vi "Func-엑셀 데이터를 그래프로 출력.vi"() -> ()   [LabVIEW 2015] (continued)
303.91\n303.93\n303.94\n303.96\n303.98\n303.99\n304.01\n304.03\n304.04\n304.06\n304.08\n304.1\n304.11\n304.13\n304.14\n304.16\n304.18\n304.19\n304.21\n304.23\n304.24\n304.26\n304.28\n304.3\n304.31\n304.33\n304.34\n304.36\n304.38\n304.39\n304.41\n304.43\n304.44\n304.46\n304.48\n304.49\n304.51\n304.53\n304.54\n304.56\n304.58\n304.59\n304.61\n304.63\n304.64\n304.66\n304.68\n304.69\n304.71\n304.73\n304.74\n304.76\n304.78\n304.79\n304.81\n304.83\n304.84\n304.86\n304.88\n304.89\n304.91\n304.93\n304.94\n304.96\n304.98\n304.99\n305.01\n305.03\n305.04\n305.06\n305.08\n305.09\n305.11\n305.13\n305.14\n305.16\n305.18\n305.19\n305.21\n305.23\n305.24\n305.26\n305.28\n305.29\n305.31\n305.33\n305.34\n305.36\n305.38\n305.39\n305.41\n305.43\n305.44\n305.46\n305.48\n305.49\n305.51\n305.53\n305.54\n305.56\n305.58\n305.59\n305.61\n305.63\n305.64\n305.66\n305.68\n305.69\n305.71\n305.73\n305.74\n305.76\n305.78\n305.79\n305.81\n305.83\n305.84\n305.86\n305.88\n305.89\n305.91\n305.93\n305.94\n305.96\n305.98\n305.99\n306.01\n306.03\n306.04\n306.06\n306.08\n306.09\n306.11\n306.13\n306.15\n306.16\n306.18\n306.19\n306.21\n306.23\n306.25\n306.26\n306.28\n306.29\n306.31\n306.33\n306.34\n306.36\n306.38\n306.39\n306.41\n306.43\n306.44\n306.46\n306.48\n306.5\n306.51\n306.53\n306.54\n306.56\n306.58\n306.6\n306.61\n306.63\n306.64\n306.66\n306.68\n306.69\n306.71\n306.73\n306.74\n306.76\n306.78\n306.79\n306.81\n306.83\n306.84\n306.86\n306.88\n306.89\n306.91\n306.93\n306.95\n306.96\n306.98\n306.99\n307.01\n307.03\n307.04\n307.06\n307.08\n307.09\n307.11\n307.13\n307.14\n307.16\n307.18\n307.2\n307.21\n307.23\n307.24\n307.26\n307.28\n307.29\n307.31\n307.33\n307.34\n307.36\n307.38\n307.39\n307.41\n307.43\n307.44\n307.46\n307.48\n307.49\n307.51\n307.53\n307.54\n307.56\n307.58\n307.59\n307.61\n307.63\n307.65\n307.66\n307.68\n307.69\n307.71\n307.73\n307.74\n307.76\n307.78\n307.79\n307.81\n307.83\n307.84\n307.86\n307.88\n307.89\n307.91\n307.93\n307.94\n307.96\n307.98\n307.99\n308.01\n308.03\n308.04\n308.06\n308.08\n308.09\n308.11\n308.13\n308.14\n308.16\n308.18\n308.19\n308.21\n308.23\n308.24\n308.26\n308.28\n308.29\n308.31\n308.33\n308.34\n308.36\n308.38\n308.39\n308.41\n308.43\n308.44\n308.46\n308.48\n308.49\n308.51\n308.53\n308.54\n308.56\n308.58\n308.59\n308.61\n308.63\n308.64\n308.66\n308.68\n308.69\n308.71\n308.73\n308.74\n308.76\n308.78\n308.79\n308.81\n308.83\n308.84\n308.86\n308.88\n308.89\n308.91\n308.93\n308.94\n308.96\n308.98\n309\n309.01\n309.03\n309.04\n309.06\n309.08\n309.09\n309.11\n309.13\n309.14\n309.16\n309.18\n309.19\n309.21\n309.23\n309.25\n309.26\n309.28\n309.29\n309.31\n309.33\n309.35\n309.36\n309.38\n309.39\n309.41\n309.43\n309.44\n309.46\n309.48\n309.49\n309.51\n309.53\n309.54\n309.56\n309.58\n309.6\n309.61\n309.63\n309.64\n309.66\n309.68\n309.7\n309.71\n309.73\n309.74\n309.76\n309.78\n309.8\n309.81\n309.83\n309.84\n309.86\n309.88\n309.89\n309.91\n309.93\n309.94\n309.96\n309.98\n309.99\n310.01\n310.03\n310.04\n310.06\n310.08\n310.09\n310.11\n310.13\n310.14\n310.16\n310.18\n310.19\n310.21\n310.23\n310.24\n310.26\n310.28\n310.3\n310.31\n310.33\n310.34\n310.36\n310.38\n310.39\n310.41\n310.43\n310.44\n310.46\n310.48\n310.49\n310.51\n310.53\n310.54\n310.56\n310.58\n310.59\n310.61\n310.63\n310.64\n310.66\n310.68\n310.69\n310.71\n310.73\n310.74\n310.76\n310.78\n310.79\n310.81\n310.83\n310.84\n310.86\n310.88\n310.89\n310.91\n310.93\n310.94\n310.96\n310.98\n310.99\n311.01\n311.03\n311.04\n311.06\n311.08\n311.09\n311.11\n311.13\n311.14\n311.16\n311.18\n311.19\n311.21\n311.23\n311.24\n311.26\n311.28\n311.29\n311.31\n311.33\n311.34\n311.36\n311.38\n311.39\n311.41\n311.43\n311.44\n311.46\n311.48\n311.49\n311.51\n311.53\n311.54\n311.56\n311.58\n311.59\n311.61\n311.63\n311.64\n311.66\n311.68\n311.69\n311.71\n311.73\n311.74\n311.76\n311.78\n311.79\n311.81\n311.83\n311.84\n311.86\n311.88\n311.89\n311.91\n311.93\n311.94\n311.96\n311.98\n311.99\n312.01\n312.03\n312.04\n312.06\n312.08\n312.1\n312.11\n312.13\n312.14\n312.16\n312.18\n312.19\n312.21\n312.23\n312.24\n312.26\n312.28\n312.29\n312.31\n312.33\n312.35\n312.36\n312.38\n312.39\n312.41\n312.43\n312.44\n312.46\n312.48\n312.49\n312.51\n312.53\n312.54\n312.56\n312.58\n312.59\n312.61\n312.63\n312.64\n312.66\n312.68\n312.7\n312.71\n312.73\n312.74\n312.76\n312.78\n312.8\n312.81\n312.83\n312.84\n312.86\n312.88\n312.89\n312.91\n312.93\n312.94\n312.96\n312.98\n312.99\n313.01\n313.03\n313.05\n313.06\n313.08\n313.09\n313.11\n313.13\n313.14\n313.16\n313.18\n313.19\n313.21\n313.23\n313.24\n313.26\n313.28\n313.29\n313.31\n313.33\n313.34\n313.36\n313.38\n313.39\n313.41\n313.43\n313.44\n313.46\n313.48\n313.49\n313.51\n313.53\n313.54\n313.56\n313.58\n313.59\n313.61\n313.63\n313.64\n313.66\n313.68\n313.69\n313.71\n313.73\n313.75\n313.76\n313.78\n313.79\n313.81\n313.83\n313.84\n313.86\n313.88\n313.89\n313.91\n313.93\n313.94\n313.96\n313.98\n313.99\n314.01\n314.03\n314.04\n314.06\n314.08\n314.09\n314.11\n314.13\n314.14\n314.16\n314.18\n314.19\n314.21\n314.23\n314.24\n314.26\n314.28\n314.29\n314.31\n314.33\n314.34\n314.36\n314.38\n314.39\n314.41\n314.43\n314.44\n314.46\n314.48\n314.49\n314.51\n314.53\n314.54\n314.56\n314.58\n314.59\n314.61\n314.63\n314.64\n314.66\n314.68\n314.69\n314.71\n314.73\n314.74\n314.76\n314.78\n314.79\n314.81\n314.83\n314.84\n314.86\n314.88\n314.89\n314.91\n314.93\n314.94\n314.96\n314.98\n314.99\n315.01\n315.03\n315.04\n315.06\n315.08\n315.09\n315.11\n315.13\n315.14\n315.16\n315.18\n315.19\n315.21\n315.23\n315.24\n315.26\n315.28\n315.29\n315.31\n315.33\n315.34\n315.36\n315.38\n315.39\n315.41\n315.43\n315.45\n315.46\n315.48\n315.49\n315.51\n315.53\n315.55\n315.56\n315.58\n315.59\n315.61\n315.63\n315.64\n315.66\n315.68\n315.69\n315.71\n315.73\n315.74\n315.76\n315.78\n315.8\n315.81\n315.83\n315.84\n315.86\n315.88\n315.9\n315.91\n315.93\n315.94\n315.96\n315.98\n315.99\n316.01\n316.03\n316.04\n316.06\n316.08\n316.09\n316.11\n316.13\n316.14\n316.16\n316.18\n316.19\n316.21\n316.23\n316.24\n316.26\n316.28\n316.29\n316.31\n316.33\n316.35\n316.36\n316.38\n316.39\n316.41\n316.43\n316.44\n316.46\n316.48\n316.49\n316.51\n316.53\n316.54\n316.56\n316.58\n316.59\n316.61\n316.63\n316.64\n316.66\n316.68\n316.7\n316.71\n316.73\n316.74\n316.76\n316.78\n316.79\n316.81\n316.83\n316.84\n316.86\n316.88\n316.89\n316.91\n316.93\n316.94\n316.96\n316.98\n316.99\n317.01\n317.03\n317.04\n317.06\n317.08\n317.09\n317.11\n317.13\n317.14\n317.16\n317.18\n317.19\n317.21\n317.23\n317.24\n317.26\n317.28\n317.29\n317.31\n317.33\n317.34\n317.36\n317.38\n317.39\n317.41\n317.43\n317.44\n317.46\n317.48\n317.49\n317.51\n317.53\n317.54\n317.56\n317.58\n317.59\n317.61\n317.63\n317.64\n317.66\n317.68\n317.69\n317.71\n317.73\n317.74\n317.76\n317.78\n317.79\n317.81\n317.83\n317.84\n317.86\n317.88\n317.89\n317.91\n317.93\n317.94\n317.96\n317.98\n317.99\n318.01\n318.03\n318.04\n318.06\n318.08\n318.09\n318.11\n318.13\n318.14\n318.16\n318.18\n318.19\n318.21\n318.23\n318.24\n318.26\n318.28\n318.3\n318.31\n318.33\n318.34\n318.36\n318.38\n318.39\n318.41\n318.43\n318.44\n318.46\n318.48\n318.49\n318.51\n318.53\n318.54\n318.56\n318.58\n318.59\n318.61\n318.63\n318.64\n318.66\n318.68\n318.69\n318.71\n318.73\n318.74\n318.76\n318.78\n318.79\n318.81\n318.83\n318.84\n318.86\n318.88\n318.9\n318.91\n318.93\n318.94\n318.96\n318.98\n319\n319.01\n319.03\n319.04\n319.06\n319.08\n319.09\n319.11\n319.13\n319.14\n319.16\n319.18\n319.19\n319.21\n319.23\n319.24\n319.26\n319.28\n319.29\n319.31\n319.33\n319.34\n319.36\n319.38\n319.39\n319.41\n319.43\n319.44\n319.46\n319.48\n319.5\n319.51\n319.53\n319.54\n319.56\n319.58\n319.59\n319.61\n319.63\n319.64\n319.66\n319.68\n319.7\n319.71\n319.73\n319.74\n319.76\n319.78\n319.8\n319.81\n319.83\n319.84\n319.86\n319.88\n319.89\n319.91\n319.93\n319.94\n319.96\n319.98\n319.99\n320.01\n320.03\n320.04\n320.06\n320.08\n320.1\n320.11\n320.13\n320.14\n320.16\n320.18\n320.19\n320.21\n320.23\n320.24\n320.26\n320.28\n320.29\n320.31\n320.33\n320.34\n320.36\n320.38\n320.39\n320.41\n320.43\n320.44\n320.46\n320.48\n320.49\n320.51\n320.53\n320.54\n320.56\n320.58\n320.59\n320.61\n320.63\n320.64\n320.66\n320.68\n320.69\n320.71\n320.73\n320.74\n320.76\n320.78\n320.79\n320.81\n320.83\n320.84\n320.86\n320.88\n320.89\n320.91\n320.93\n320.94\n320.96\n320.98\n320.99\n321.01\n321.03\n321.04\n321.06\n321.08\n321.09\n321.11\n321.13\n321.14\n321.16\n321.18\n321.19\n321.21\n321.23\n321.24\n321.26\n321.28\n321.3\n321.31\n321.33\n321.34\n321.36\n321.38\n321.39\n321.41\n321.43\n321.44\n321.46\n321.48\n321.49\n321.51\n321.53\n321.54\n321.56\n321.58\n321.59\n321.61\n321.63\n321.65\n321.66\n321.68\n321.69\n321.71\n321.73\n321.75\n321.76\n321.78\n321.79\n321.81\n321.83\n321.84\n321.86\n321.88\n321.89\n321.91\n321.93\n321.94\n321.96\n321.98\n322\n322.01\n322.03\n322.04\n322.06\n322.08\n322.1\n322.11\n322.13\n322.14\n322.16\n322.18\n322.19\n322.21\n322.23\n322.24\n322.26\n322.28\n322.29\n322.31\n322.33\n322.35\n322.36\n322.38\n322.39\n322.41\n322.43\n322.44\n322.46\n322.48\n322.49\n322.51\n322.53\n322.54\n322.56\n322.58\n322.6\n322.61\n322.63\n322.64\n322.66\n322.68\n322.69\n322.71\n322.73\n322.74\n322.76\n322.78\n322.79\n322.81\n322.83\n322.84\n322.86\n322.88\n322.89\n322.91\n322.93\n322.94\n322.96\n322.98\n322.99\n323.01\n323.03\n323.04\n323.06\n323.08\n323.09\n323.11\n323.13\n323.14\n323.16\n323.18\n323.19\n323.21\n323.23\n323.24\n323.26\n323.28\n323.29\n323.31\n323.33\n323.34\n323.36\n323.38\n323.39\n323.41\n323.43\n323.44\n323.46\n323.48\n323.49\n323.51\n323.53\n323.54\n323.56\n323.58\n323.59\n323.61\n323.63\n323.64\n323.66\n323.68\n323.69\n323.71\n323.73\n323.74\n323.76\n323.78\n323.79\n323.81\n323.83\n323.84\n323.86\n323.88\n323.89\n323.91\n323.93\n323.94\n323.96\n323.98\n323.99\n324.01\n324.03\n324.04\n324.06\n324.08\n324.09\n324.11\n324.13\n324.14\n324.16\n324.18\n324.19\n324.21\n324.23\n324.24\n324.26\n324.28\n324.29\n324.31\n324.33\n324.34\n324.36\n324.38\n324.39\n324.41\n324.43\n324.44\n324.46\n324.48\n324.49\n324.51\n324.53\n324.54\n324.56\n324.58\n324.59\n324.61\n324.63\n324.64\n324.66\n324.68\n324.69\n324.71\n324.73\n324.75\n324.76\n324.78\n324.79\n324.81\n324.83\n324.85\n324.86\n324.88\n324.89\n324.91\n324.93\n324.94\n324.96\n324.98\n324.99\n325.01\n325.03\n325.04\n325.06\n325.08\n325.1\n325.11\n325.13\n325.14\n325.16\n325.18\n325.2\n325.21\n325.23\n325.24\n325.26\n325.28\n325.29\n325.31\n325.33\n325.34\n325.36\n325.38\n325.39\n325.41\n325.43\n325.45\n325.46\n325.48\n325.49\n325.51\n325.53\n325.55\n325.56\n325.58\n325.59\n325.61\n325.63\n325.64\n325.66\n325.68\n325.7\n325.71\n325.73\n325.74\n325.76\n325.78\n325.8\n325.81\n325.83\n325.84\n325.86\n325.88\n325.9\n325.91\n325.93\n325.94\n325.96\n325.98\n325.99\n326.01\n326.03\n326.04\n326.06\n326.08\n326.09\n326.11\n326.13\n326.14\n326.16\n326.18\n326.19\n326.21\n326.23\n326.24\n326.26\n326.28\n326.29\n326.31\n326.33\n326.34\n326.36\n326.38\n326.39\n326.41\n326.43\n326.44\n326.46\n326.48\n326.49\n326.51\n326.53\n326.54\n326.56\n326.58\n326.59\n326.61\n326.63\n326.64\n326.66\n326.68\n326.69\n326.71\n326.73\n326.74\n326.76\n326.78\n326.79\n326.81\n326.83\n326.84\n326.86\n326.88\n326.89\n326.91\n326.93\n326.94\n326.96\n326.98\n326.99\n327.01\n327.03\n327.04\n327.06\n327.08\n327.09\n327.11\n327.13\n327.14\n327.16\n327.18\n327.19\n327.21\n327.23\n327.24\n327.26\n327.28\n327.29\n327.31\n327.33\n327.34\n327.36\n327.38\n327.39\n327.41\n327.43\n327.44\n327.46\n327.48\n327.49\n327.51\n327.53\n327.54\n327.56\n327.58\n327.59\n327.61\n327.63\n327.64\n327.66\n327.68\n327.69\n327.71\n327.73\n327.74\n327.76\n327.78\n327.79\n327.81\n327.83\n327.85\n327.86\n327.88\n327.89\n327.91\n327.93\n327.94\n327.96\n327.98\n327.99\n328.01\n328.03\n328.04\n328.06\n328.08\n328.09\n328.11\n328.13\n328.14\n328.16\n328.18\n328.2\n328.21\n328.23\n328.24\n328.26\n328.28\n328.3\n328.31\n328.33\n328.34\n328.36\n328.38\n328.39\n328.41\n328.43\n328.44\n328.46\n328.48\n328.49\n328.51\n328.53\n328.55\n328.56\n328.58\n328.59\n328.61\n328.63\n328.64\n328.66\n328.68\n328.69\n328.71\n328.73\n328.74\n328.76\n328.78\n328.8\n328.81\n328.83\n328.84\n328.86\n328.88\n328.9\n328.91\n328.93\n328.94\n328.96\n328.98\n328.99\n329.01\n329.03\n329.04\n329.06\n329.08\n329.1\n329.11\n329.13\n329.15\n329.16\n329.18\n329.19\n329.21\n329.23\n329.24\n329.26\n329.28\n329.29\n329.31\n329.33\n329.34\n329.36\n329.38\n329.39\n329.41\n329.43\n329.45\n329.46\n329.48\n329.49\n329.51\n329.53\n329.54\n329.56\n329.58\n329.59\n329.61\n329.63\n329.64\n329.66\n329.68\n329.69\n329.71\n329.73\n329.74\n329.76\n329.78\n329.79\n329.81\n329.83\n329.84\n329.86\n329.88\n329.89\n329.91\n329.93\n329.94\n329.96\n329.98\n329.99\n330.01\n330.03\n330.04\n330.06\n330.08\n330.09\n330.11\n330.13\n330.14\n330.16\n330.18\n330.19\n330.21\n330.23\n330.24\n330.26\n330.28\n330.29\n330.31\n330.33\n330.34\n330.36\n330.38\n330.39\n330.41\n330.43\n330.44\n330.46\n330.48\n330.49\n330.51\n330.53\n330.54\n330.56\n330.58\n330.6\n330.61\n330.63\n330.64\n330.66\n330.68\n330.69\n330.71\n330.73\n330.74\n330.76\n330.78\n330.79\n330.81\n330.83\n330.84\n330.86\n330.88\n330.89\n330.91\n330.93\n330.95\n330.96\n330.98\n330.99\n331.01\n331.03\n331.05\n331.06\n331.08\n331.09\n331.11\n331.13\n331.14\n331.16\n331.18\n331.19\n331.21\n331.23\n331.24\n331.26\n331.28\n331.3\n331.31\n331.33\n331.34\n331.36\n331.38\n331.4\n331.41\n331.43\n331.44\n331.46\n331.48\n331.49\n331.51\n331.53\n331.54\n331.56\n331.58\n331.59\n331.61\n331.63\n331.65\n331.66\n331.68\n331.69\n331.71\n331.73\n331.74\n331.76\n331.78\n331.79\n331.81\n331.83\n331.84\n331.86\n331.88\n331.9\n331.91\n331.93\n331.94\n331.96\n331.98\n332\n332.01\n332.03\n332.04\n332.06\n332.08\n332.09\n332.11\n332.13\n332.14\n332.16\n332.18\n332.19\n332.21\n332.23\n332.25\n332.26\n332.28\n332.29\n332.31\n332.33\n332.34\n332.36\n332.38\n332.39\n332.41\n332.43\n332.45\n332.46\n332.48\n332.49\n332.51\n332.53\n332.54\n332.56\n332.58\n332.59\n332.61\n332.63\n332.64\n332.66\n332.68\n332.69\n332.71\n332.73\n332.74\n332.76\n332.78\n332.79\n332.81\n332.83\n332.84\n332.86\n332.88\n332.89\n332.91\n332.93\n332.94\n332.96\n332.98\n332.99\n333.01\n333.03\n333.04\n333.06\n333.08\n333.09\n333.11\n333.13\n333.14\n333.16\n333.18\n333.19\n333.21\n333.23\n333.24\n333.26\n333.28\n333.29\n333.31\n333.33\n333.34\n333.36\n333.38\n333.39\n333.41\n333.43\n333.44\n333.46\n333.48\n333.49\n333.51\n333.53\n333.54\n333.56\n333.58\n333.59\n333.61\n333.63\n333.64\n333.66\n333.68\n333.69\n333.71\n333.73\n333.74\n333.76\n333.78\n333.79\n333.81\n333.83\n333.84\n333.86\n333.88\n333.89\n333.91\n333.93\n333.94\n333.96\n333.98\n333.99\n334.01\n334.03\n334.05\n334.06\n334.08\n334.09\n334.11\n334.13\n334.14\n334.16\n334.18\n334.19\n334.21\n334.23\n334.24\n334.26\n334.28\n334.29\n334.31\n334.33\n334.34\n334.36\n334.38\n334.4\n334.41\n334.43\n334.44\n334.46\n334.48\n334.5\n334.51\n334.53\n334.54\n334.56\n334.58\n334.59\n334.61\n334.63\n334.64\n334.66\n334.68\n334.69\n334.71\n334.73\n334.75\n334.76\n334.78\n334.79\n334.81\n334.83\n334.85\n334.86\n334.88\n334.89\n334.91\n334.93\n334.94\n334.96\n334.98\n334.99\n335.01\n335.03\n335.04\n335.06\n335.08\n335.1\n335.11\n335.13\n335.14\n335.16\n335.18\n335.2\n335.21\n335.23\n335.24\n335.26\n335.28\n335.3\n335.31\n335.33\n335.34\n335.36\n335.38\n335.39\n335.41\n335.43\n335.45\n335.46\n335.48\n335.49\n335.51\n335.53\n335.54\n335.56\n335.58\n335.59\n335.61\n335.63\n335.64\n335.66\n335.68\n335.69\n335.71\n335.73\n335.74\n335.76\n335.78\n335.79\n335.81\n335.83\n335.84\n335.86\n335.88\n335.89\n335.91\n335.93\n335.94\n335.96\n335.98\n335.99\n336.01\n336.03\n336.04\n336.06\n336.08\n336.09\n336.11\n336.13\n336.14\n336.16\n336.18\n336.19\n336.21\n336.23\n336.24\n336.26\n336.28\n336.29\n336.31\n336.33\n336.34\n336.36\n336.38\n336.39\n336.41\n336.43\n336.44\n336.46\n336.48\n336.49\n336.51\n336.53\n336.54\n336.56\n336.58\n336.59\n336.61\n336.63\n336.64\n336.66\n336.68\n336.69\n336.71\n336.73\n336.74\n336.76\n336.78\n336.79\n336.81\n336.83\n336.84\n336.86\n336.88\n336.89\n336.91\n336.93\n336.94\n336.96\n336.98\n336.99\n337.01\n337.03\n337.04\n337.06\n337.08\n337.09\n337.11\n337.13\n337.14\n337.16\n337.18\n337.19\n337.21\n337.23\n337.25\n337.26\n337.28\n337.29\n337.31\n337.33\n337.34\n337.36\n337.38\n337.39\n337.41\n337.43\n337.44\n337.46\n337.48\n337.5\n337.51\n337.53\n337.54\n337.56\n337.58\n337.6\n337.61\n337.63\n337.64\n337.66\n337.68\n337.69\n337.71\n337.73\n337.74\n337.76\n337.78\n337.79\n337.81\n337.83\n337.85\n337.86\n337.88\n337.89\n337.91\n337.93\n337.95\n337.96\n337.98\n337.99\n338.01\n338.03\n338.04\n338.06\n338.08\n338.1\n338.11\n338.13\n338.14\n338.16\n338.18\n338.2\n338.21\n338.23\n338.24\n338.26\n338.28\n338.29\n338.31\n338.33\n338.34\n338.36\n338.38\n338.39\n338.41\n338.43\n338.44\n338.46\n338.48\n338.49\n338.51\n338.53\n338.55\n338.56\n338.58\n338.59\n338.61\n338.63\n338.64\n338.66\n338.68\n338.69\n338.71\n338.73\n338.74\n338.76\n338.78\n338.79\n338.81\n338.83\n338.84\n338.86\n338.88\n338.89\n338.91\n338.93\n338.94\n338.96\n338.98\n338.99\n339.01\n339.03\n339.04\n339.06\n339.08\n339.09\n339.11\n339.13\n339.14\n339.16\n339.18\n339.19\n339.21\n339.23\n339.24\n339.26\n339.28\n339.29\n339.31\n339.33\n339.34\n339.36\n339.38\n339.39\n339.41\n339.43\n339.44\n339.46\n339.48\n339.49\n339.51\n339.53\n339.54\n339.56\n339.58\n339.59\n339.61\n339.63\n339.64\n339.66\n339.68\n339.69\n339.71\n339.73\n339.74\n339.76\n339.78\n339.79\n339.81\n339.83\n339.84\n339.86\n339.88\n339.89\n339.91\n339.93\n339.94\n339.96\n339.98\n339.99\n340.01\n340.03\n340.04\n340.06\n340.08\n340.09\n340.11\n340.13\n340.14\n340.16\n340.18\n340.19\n340.21\n340.23\n340.24\n340.26\n340.28\n356.83\n357\n357.16\n357.33\n357.5\n357.66\n357.83\n358\n358.16\n358.33\n358.5\n358.66\n358.83\n359\n359.16\n359.33\n359.5\n359.67\n359.83\n360\n360.16\n360.33\n360.51\n360.67\n360.84\n361.01\n361.17\n361.34\n361.51\n361.67\n361.84\n362.01\n362.17\n362.34\n362.51\n362.67\n362.84\n363.01\n363.17\n363.34\n363.51\n363.67\n363.84\n364.01\n364.17\n364.34\n364.51\n364.67\n364.84\n365.01\n365.17\n365.34\n365.51\n365.67\n365.84\n366.01\n366.17\n366.34\n366.51\n366.67\n366.84\n367.01\n367.18\n367.35\n367.51\n367.68\n367.85\n368.01\n368.18\n368.35\n368.52\n368.68\n368.85\n369.01\n369.18\n369.35\n369.51\n369.68\n369.85\n370.01\n370.18\n370.35\n370.51\n370.68\n370.85\n371.01\n371.18\n371.35\n371.51\n371.68\n371.85\n372.01\n372.18\n372.35\n372.51\n372.68\n372.85\n373.01\n373.18\n373.35\n373.51\n373.68\n373.85\n374.01\n374.18\n374.35\n374.51\n374.68\n374.85\n375.01\n375.18\n375.35\n375.52\n375.68\n375.85\n376.01\n376.18\n376.35\n376.51\n376.68\n376.85\n377.01\n377.18\n377.35\n377.51\n377.68\n377.85\n378.01\n378.18\n378.35\n378.51\n378.68\n378.85\n379.01\n379.2\n379.35\n379.51\n379.68\n379.85\n380.01\n380.2\n380.37\n380.53\n380.7\n380.85\n381.03\n381.2\n381.37\n381.53\n381.7\n381.87\n382.03\n382.2\n382.37\n382.53\n382.7\n382.87\n383.04\n383.19\n383.36\n383.52\n383.69\n383.86\n384.02\n384.19\n384.36\n384.52\n384.69\n384.86\n385.02\n385.19\n385.36\n385.52\n385.69\n385.86\n386.02\n386.19\n386.36\n386.52\n386.69\n386.86\n387.02\n387.19\n387.36\n387.52\n387.69\n387.86\n388.02\n388.19\n388.36\n388.52\n388.69\n388.86\n389.02\n389.19\n389.36\n389.52\n389.69\n389.86\n390.02\n390.19\n390.36\n390.52\n390.69\n390.86\n391.02\n391.19\n391.36\n391.52\n391.69\n391.86\n392.02\n392.19\n392.36\n392.52\n392.69\n392.86\n393.02\n393.19\n393.36\n393.52\n393.69\n393.86\n394.02\n394.19\n394.36\n394.52\n394.69\n394.86\n395.02\n395.19\n395.36\n395.52\n395.69\n395.86\n396.02\n396.19\n396.36\n396.51\n396.51\n396.53\n396.54\n396.56\n396.58\n396.59\n396.61\n396.63\n396.64\n396.66\n396.68\n396.69\n396.71\n396.73\n396.75\n396.76\n396.78\n396.79\n396.81\n396.83\n396.84\n396.86\n396.88\n396.89\n396.91\n396.93\n396.94\n396.96\n396.98\n396.99\n397.01\n397.03\n397.04\n397.06\n397.08\n397.1\n397.11\n397.13\n397.14\n397.16\n397.18\n397.2\n397.21\n397.23\n397.24\n397.26\n397.28\n397.29\n397.31\n397.33\n397.34\n397.36\n397.38\n397.39\n397.41\n397.43\n397.45\n397.46\n397.48\n397.49\n397.51\n397.53\n397.54\n397.56\n397.58\n397.59\n397.61\n397.63\n397.64\n397.66\n397.68\n397.69\n397.71\n397.73\n397.74\n397.76\n397.78\n397.79\n397.81\n397.83\n397.84\n397.86\n397.88\n397.89\n397.91\n397.93\n397.94\n397.96
